vi "Timestamp to Datetime.vi"(11 "Time Stamp":timestamp format="%<%x %.3X>T") -> (3 "date/time string":string)   [LabVIEW 2021, in "EDT SQLite+.lvlib"]
uses:
  EDT SQLite+.lvlib
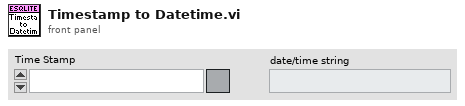
[diagram p1: front panel]
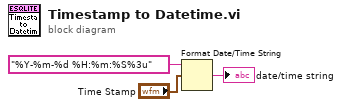
[diagram p0: block diagram]
diagram:
  n1 = Format Date/Time String(time format string (%c)="%Y-%m-%d %H:%m:%S%3u", seconds (now)="Time Stamp") -> (date/time string=→"date/time string":string)  [unwired: 1 in]
